vi "MAIL.vi"(9 "寄送":bool, 10 "內容":string, 11 "標題":string) -> ()   [LabVIEW 2017]
uses:
  <vilib>/smtpClient/Set Message Text.vi
  <vilib>/smtpClient/LabVIEWSMTPClient.lvlib
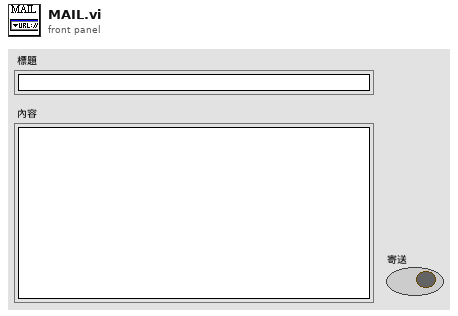
[diagram p1: front panel]
types:
  T1 = typedef "LabVIEWSMTPClient.lvlib/SmtpClientHandle.ctl" = refnum<k1>
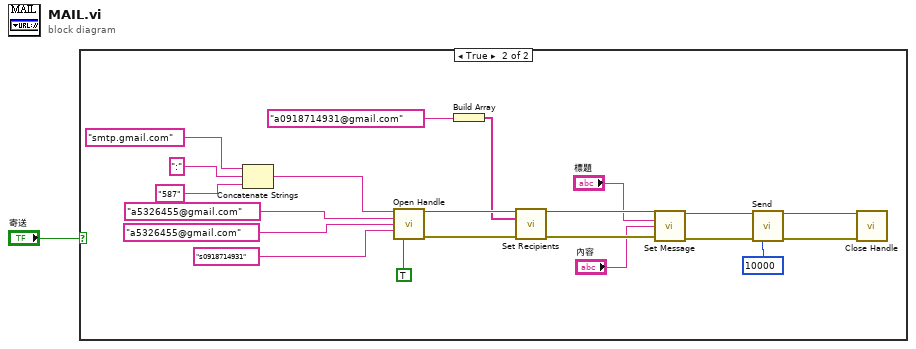
[diagram p0: block diagram]
diagram:
  n1 = case shown="True" "寄送" {
    frame False {
    }
    frame True {
      n2 = Concatenate Strings("smtp.gmail.com" ("subject"), ":" ("subject"), "587" ("subject")) -> (w7:string)
      n3 = call <vilib>:"Open Handle.vi"("server address"=w7, "from"="a5326455@gmail.com" ("subject"), "username"="a5326455@gmail.com" ("subject"), "password"="s0918714931" ("subject"), "use TLS (false)"=TRUE) -> ("handle out"=w15:T1, "error out"=w14:errorcluster)  [unwired: 9 in]
      n4 = Build Array("a0918714931@gmail.com" ("subject")) -> (w11:string[])
      n5 = call <vilib>:"Set Recipients.vi"("handle in"=w15, "to"=w11, "error in (no error)"=w14) -> ("handle out"=w17:T1, "error out"=w16:errorcluster)  [unwired: 11 in]
      n6 = call-poly <vilib>:"Set Message.vi"("handle in"=w17, "subject"="標題", "plain text message"="內容", "error in (no error)"=w16) -> ("handle out"=w19:T1, "error out"=w18:errorcluster)  [unwired: 10 in]
      n7 = call <vilib>:"Send.vi"("handle in"=w19, "error in (no error)"=w18, "timeout in ms (10000)"=10000) -> ("handle out"=w22:T1, "error out"=w21:errorcluster)  [unwired: 10 in, 1 out]
      n8 = call <vilib>:"Close Handle.vi"("handle in"=w22, "error in (no error)"=w21) -> ()  [unwired: 12 in, 2 out]
    }
  }
